vi "Close.vi"(8 "error in":errorcluster, 11 "host in":refnum<class "LIA Host Interface FPGA.lvclass">) -> (0 "error out":errorcluster, 3 "host out":refnum<class "LIA Host Interface FPGA.lvclass">)   [LabVIEW 2017, in "LIA Host Interface FPGA.lvclass"]
uses:
  LIA Host Interface FPGA.lvclass
  LIA Host Interface FPGA.lvclass/LIA Host Interface FPGA.ctl
  <vilib>/FPGAPlugInAG/Dynamic/niLvFpga_Close_Dynamic.vi
  <vilib>/rvi/interface/nirviCloseFPGA/nirviCloseFPGA.xnode
  host/Lock-In Amplifier Example Host.lvlib
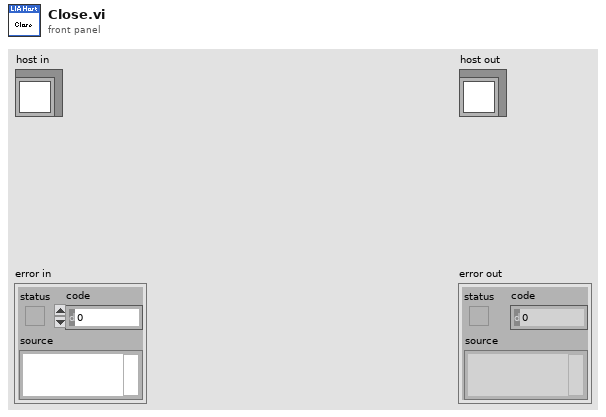
[diagram p1: front panel]
types:
  T1 = typedef "LIA Host Interface Desktop.lvclass/session data.ctl" = cluster{"fpga session":refnum<k20>, "record length":u32[]}
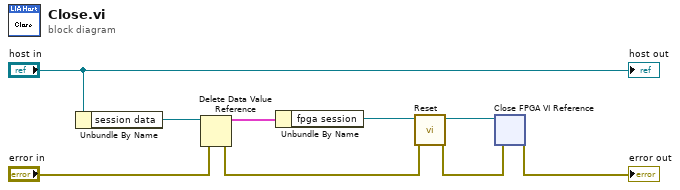
[diagram p0: block diagram]
diagram:
  n1 = Unbundle By Name("host in") -> ("session data"=w8:refnum<data-value>)
  n2 = Delete Data Value Reference(data value reference=w8, error in="error in") -> (data value=w7:T1, error out=w4:errorcluster)
  n3 = Unbundle By Name(w7) -> ("fpga session"=w5:refnum<k20>)
  n4 = call "Reset.vi"("error in"=w4, "fpga session in"=w5) -> ("error out"=w2:errorcluster, "fpga session out"=w3:refnum<k20>)  [unwired: 8 in]
  n5 = xnode "Close FPGA VI Reference"("FPGA VI Reference In"=w3, "error in"=w2) -> ("error out"=→"error out":errorcluster)
  "host out" <- "host in"
